vi "array solution.vi"() -> ()   [LabVIEW 2018]
panel:
  out "Outcome":dbl[](array[numeric])
  in  "Array":dbl[](array[numeric])
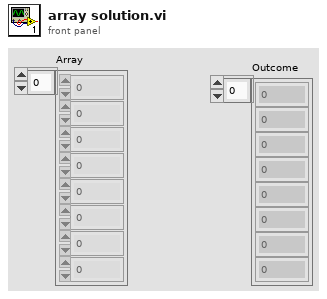
[diagram p1: front panel]
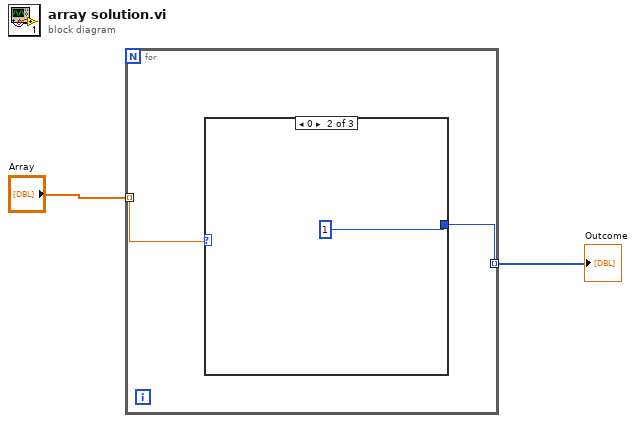
[diagram p0: block diagram]
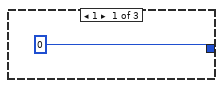
[diagram p2: hidden frame]
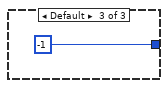
[diagram p3: hidden frame]
diagram:
  n1 = for {
    tunnel: "Array" -> [w4] mode=indexing
    tunnel: [w3] -> w1 mode=indexing
    n2 = case shown="0" w4 {
      tunnel: [0 1 -1] -> w3
      frame 1 {
      }
      frame 0 {
      }
      frame Default {
      }
    }
  }
  "Outcome" <- w1
